vi "ConvertFalconDriveEncoders.vi"(0 "Shifter State":T1(ring), 7 "Distance (Raw Sensor Units)":i32, 11 "Velocity (Raw Sensor Units per 100 ms)":i32, 12 "Shift Time Threshold (ms)":u32, 13 "Latched Shift Time (ms)":u32, 14 "Latched Velocity (ft/s)":dbl) -> (4 "Distance (in)":dbl, 15 "Velocity (ft/s)":dbl)   [LabVIEW 2019]
doc: "This VI converts the raw Falcon 500/Talon FX encoder postion and velocity data into units of inches and feet per second, respectively. Handles low and high gear ratios."
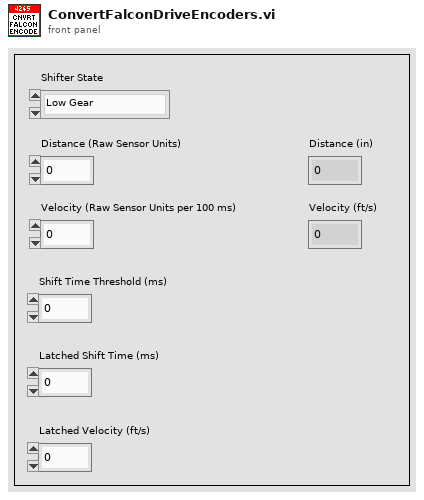
[diagram p1: front panel]
types:
  T1 = enum16{"Low Gear", "High Gear", "Transiting", "Unknown", "Force Low Gear"}
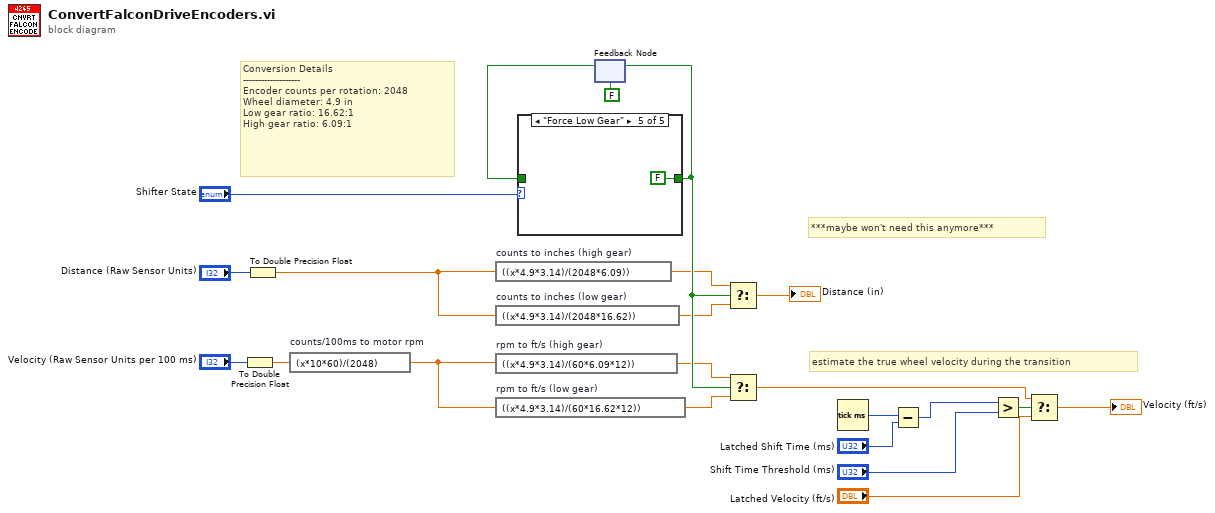
[diagram p0: block diagram]
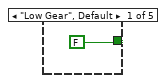
[diagram p2: hidden frame]
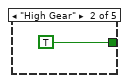
[diagram p3: hidden frame]
diagram:
  # "estimate the true wheel velocity during the transition"
  # "***maybe won't need this anymore***"
  # "Conversion Details\n-------------------\nEncoder counts per rotation: 2048\nWheel diameter: 4.9 in\nLow gear ratio: 16.62:1\nHigh gear ratio: 6.09:1"
  n1 = To Double Precision Float(number="Velocity (Raw Sensor Units per 100 ms)") -> (double precision float=w17:dbl)
  n2 = To Double Precision Float(number="Distance (Raw Sensor Units)") -> (double precision float=w16:dbl)
  n3 = expression code="(x*10*60)/(2048)" "counts/100ms to motor rpm"(w17) -> (w9:dbl)
  n4 = expression code="((x*4.9*3.14)/(2048*6.09))" "counts to inches (high gear)"(w16) -> (w12:dbl)
  n5 = expression code="((x*4.9*3.14)/(2048*16.62))" "counts to inches (low gear)"(w16) -> (w14:dbl)
  n6 = expression code="((x*4.9*3.14)/(60*6.09*12))" "rpm to ft/s (high gear)"(w9) -> (w10:dbl)
  n7 = expression code="((x*4.9*3.14)/(60*16.62*12))" "rpm to ft/s (low gear)"(w9) -> (w11:dbl)
  n8 = feedback #1(FALSE) -> (w20:bool)
  n9 = case shown="\"Force Low Gear\"" "Shifter State" {
    tunnel: [FALSE TRUE w25 w26 FALSE] -> w22
    tunnel: w20 -> [_ _ w25 w26 _]
    frame "Low Gear", Default {
    }
    frame "High Gear" {
    }
    frame "Transiting" {
    }
    frame "Unknown" {
    }
    frame "Force Low Gear" {
    }
  }
  n10 = feedback-in #1(w22) -> ()
  n11 = Select(t=w12, s=w22, f=w14) -> (s? t:f=→"Distance (in)":dbl)
  n12 = Select(t=w10, s=w22, f=w11) -> (s? t:f=w6:dbl)
  n13 = Tick Count (ms)() -> (millisecond timer value=w4:u32)
  n14 = Subtract(x=w4, y="Latched Shift Time (ms)") -> (x-y=w3:u32)
  n15 = Greater?(x=w3, y="Shift Time Threshold (ms)") -> (0:w8:bool)
  n16 = Select(t=w6, s=w8, f="Latched Velocity (ft/s)") -> (s? t:f=→"Velocity (ft/s)":dbl)
